vi "Parallel while loops.vi"() -> ()   [LabVIEW 2015]
panel:
  out "Chart 2":dbl(graph)
  out "Chart 1":dbl(graph)
  in  "stop":bool
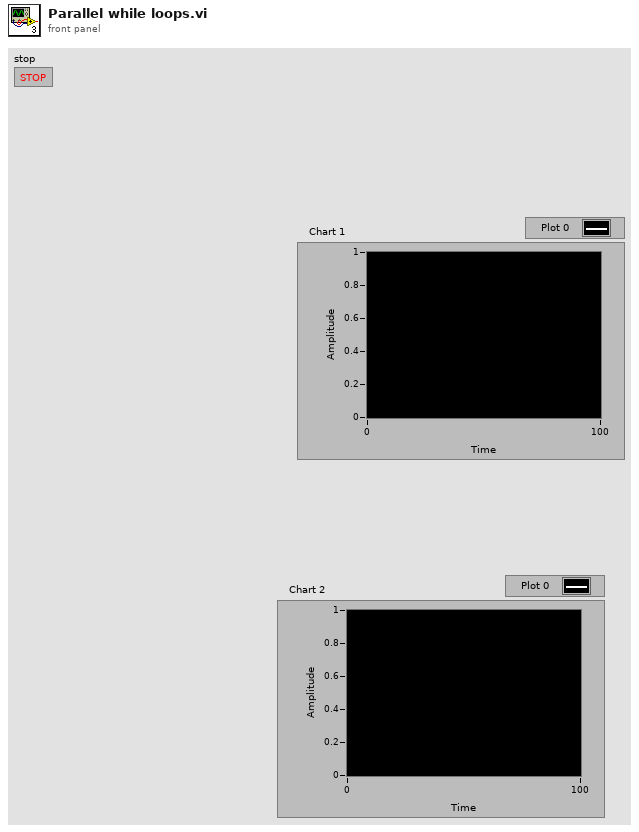
[diagram p1: front panel]
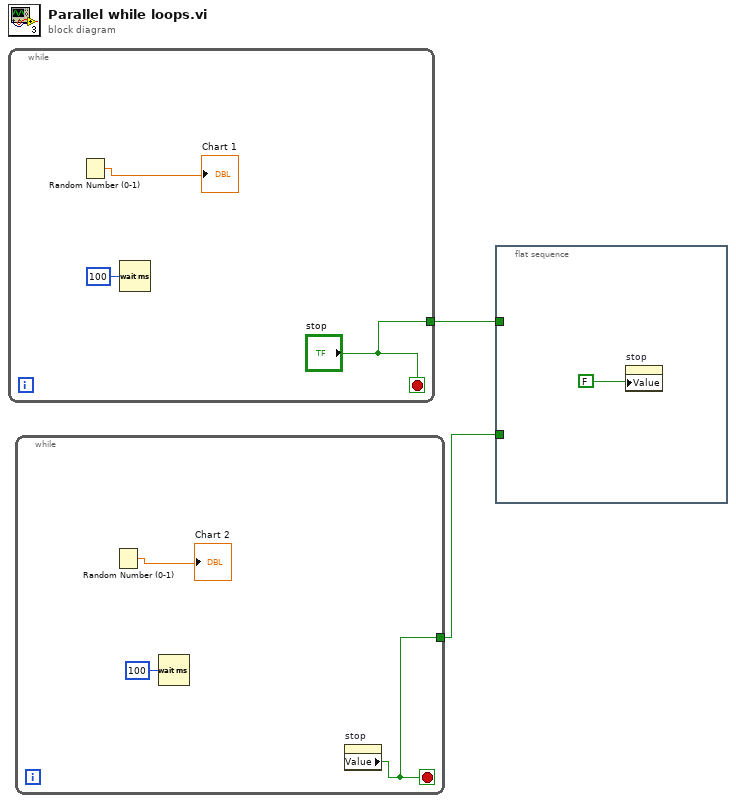
[diagram p0: block diagram]
diagram:
  n1 = while {
    tunnel: ["stop"] -> w2
    stop <- "stop" stop-if-true
    n2 = Random Number (0-1)() -> (number: 0 to 1=→"Chart 1":dbl)
    n3 = Wait (ms)(milliseconds to wait=u32 100) -> ()  [unwired: 1 out]
  }
  n4 = while {
    tunnel: [w6] -> w1
    stop <- w6 stop-if-true
    n5 = Random Number (0-1)() -> (number: 0 to 1=→"Chart 2":dbl)
    n6 = Wait (ms)(milliseconds to wait=u32 100) -> ()  [unwired: 1 out]
    n7 = property on="stop" class="Bool (strict)"() -> ("Value"=w6:bool)  [unwired: 2 in, 2 out]
  }
  n8 = flat-sequence {
    tunnel: w2 -> [_]
    tunnel: w1 -> [_]
    frame #0 {
      n9 = property on="stop" class="Bool (strict)"("Value"=FALSE) -> ()  [unwired: 2 in, 2 out]
    }
  }
